vi "process_averager_imaq.vi"() -> ()   [LabVIEW 2011, in "Fiberscope_library.lvlib"]
uses:
  Fiberscope_library.lvlib
  typedefs/control_process_state_enum.ctl
  typedefs/control_process_state_cluster.ctl
  typedefs/feedback_from_process_enum.ctl
  typedefs/feedback_to_watchdog.ctl
  <vilib>/vision/Image Controls.llb/IMAQ Image.ctl
  typedefs/element_imaq_images_cluster.ctl
  <vilib>/vision/NI_Vision_Development_Module.lvlib
panel:
  out "Averages per frame":u8
  out "Average":u8
  out "error out":errorcluster
  in  "error in":errorcluster
  # "of"
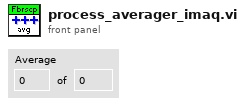
[diagram p1: front panel]
types:
  T1 = typedef "Fiberscope_library.lvlib/element_imaq_images_cluster.ctl" = cluster{"Images":T2[], "#channels":i32, "Last element?":bool}
  T2 = typedef "IMAQ Image.ctl" = refnum<image>
  T3 = typedef "Fiberscope_library.lvlib/feedback_to_watchdog.ctl" = cluster{"Feedback_from_process_enum":T4, "Process_name":string}
  T4 = typedef "Fiberscope_library.lvlib/feedback_from_process_enum.ctl" = enum16{"Has_initialised", "Changed_parameters", "Has_started", "Has_stopped", "Has_quitted", "Is_running", "Has_finished", "Custom"}
  T5 = typedef "Fiberscope_library.lvlib/control_process_state_cluster.ctl" = cluster{"Control_process_state_enum":T6, "variant":variant}
  T6 = typedef "Fiberscope_library.lvlib/control_process_state_enum.ctl" = enum16{"Init", "Quit", "Start", "Stop", "Change_parameters", "Running", "Finish", "Custom"}
  T7 = typedef "Image Type" = u32
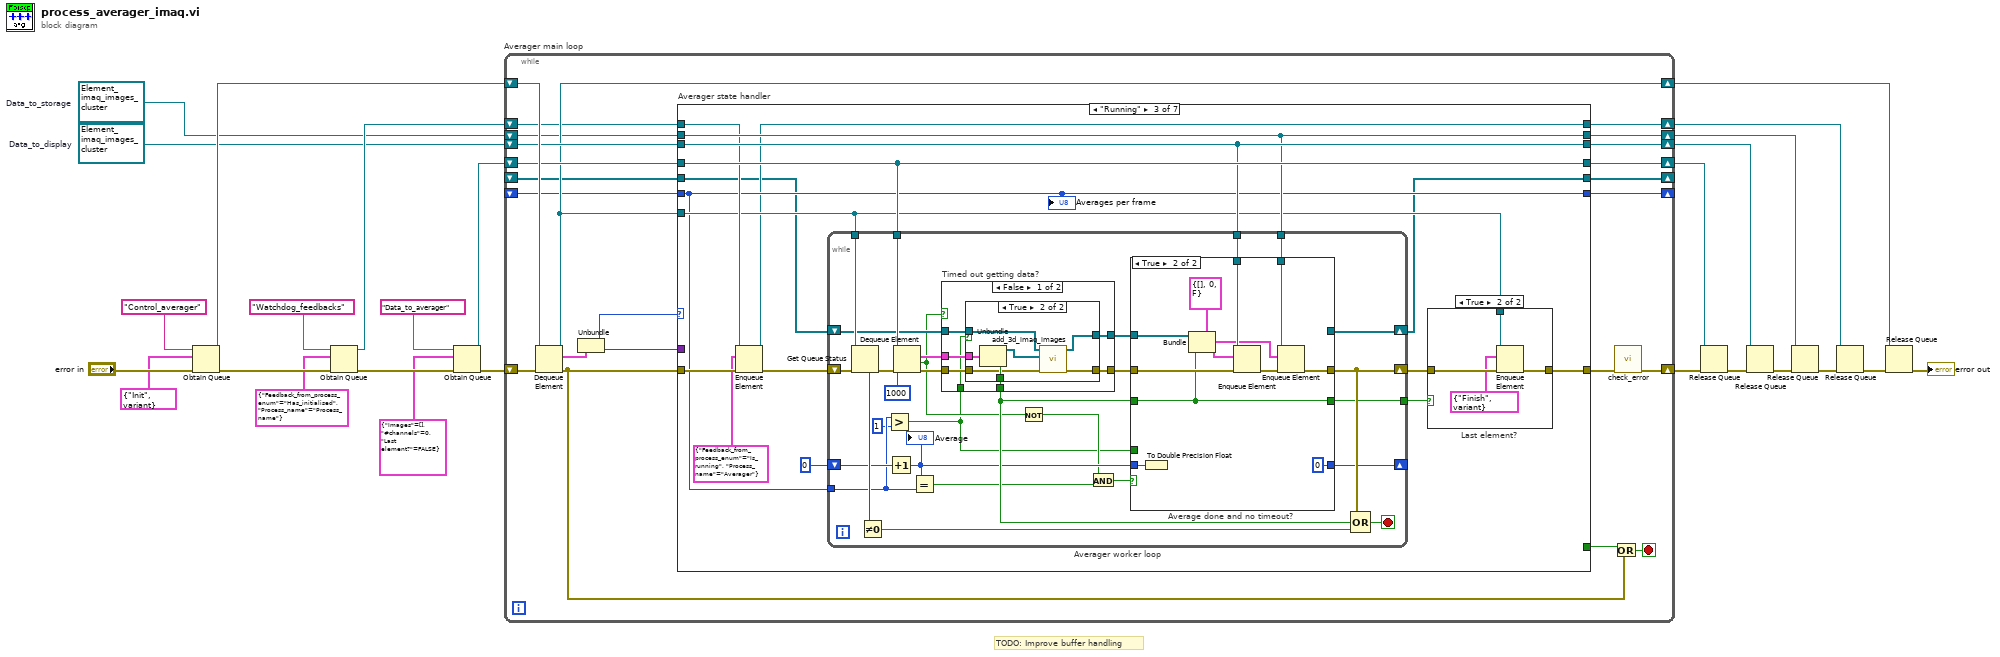
[diagram p0: block diagram]
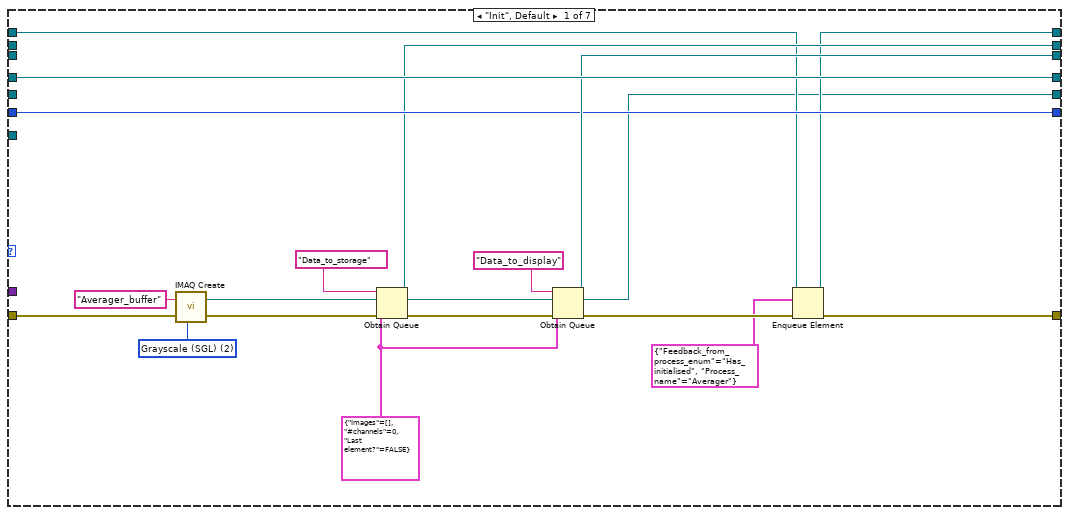
[diagram p2: hidden frame]
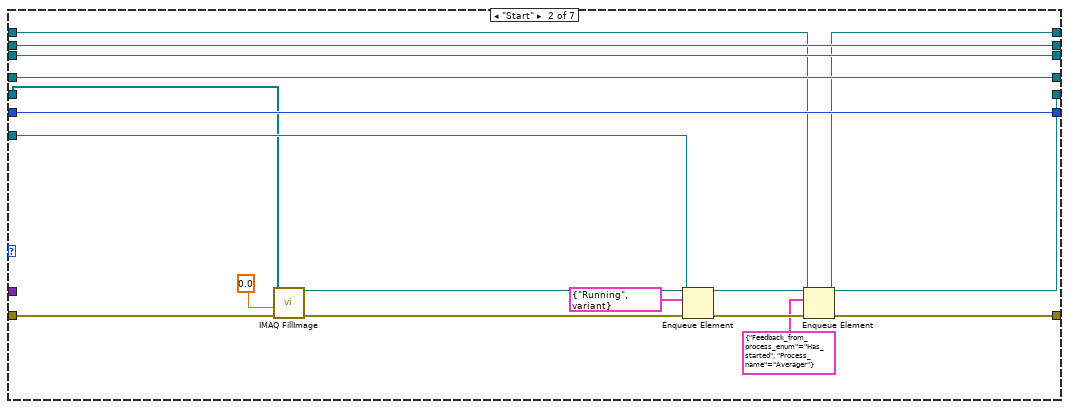
[diagram p3: hidden frame]
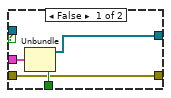
[diagram p6: hidden frame]
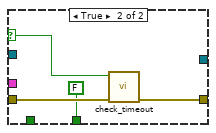
[diagram p7: hidden frame]
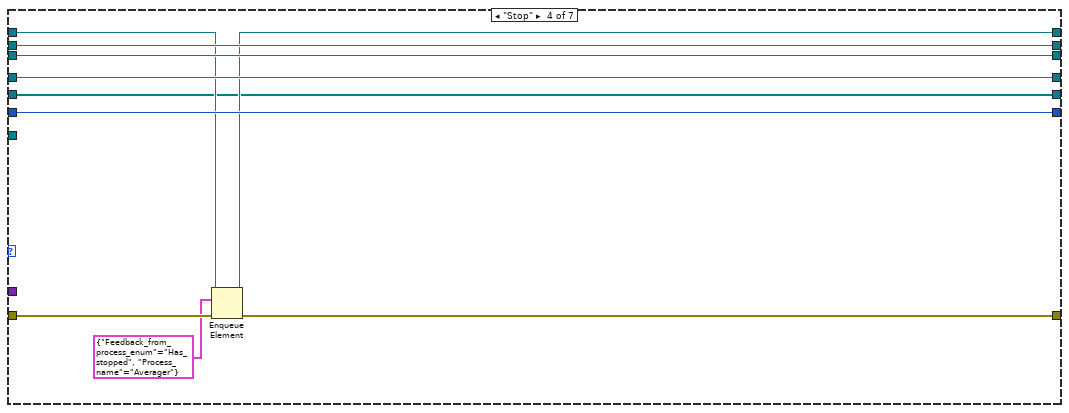
[diagram p8: hidden frame]
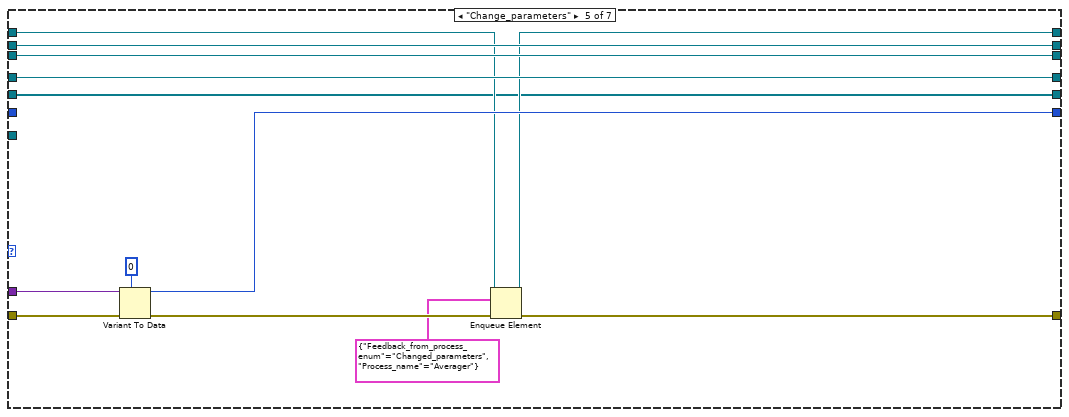
[diagram p9: hidden frame]
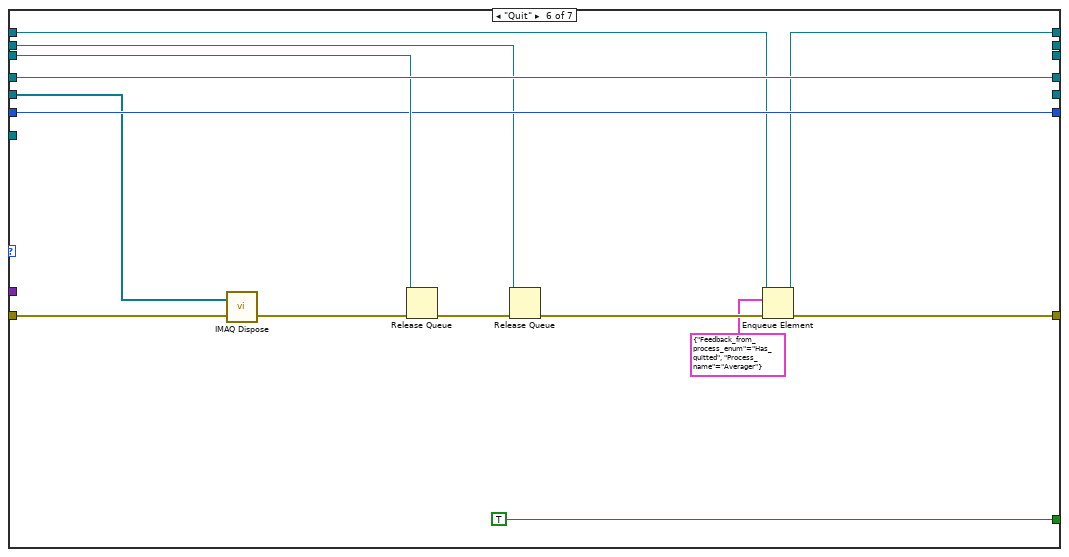
[diagram p10: hidden frame]
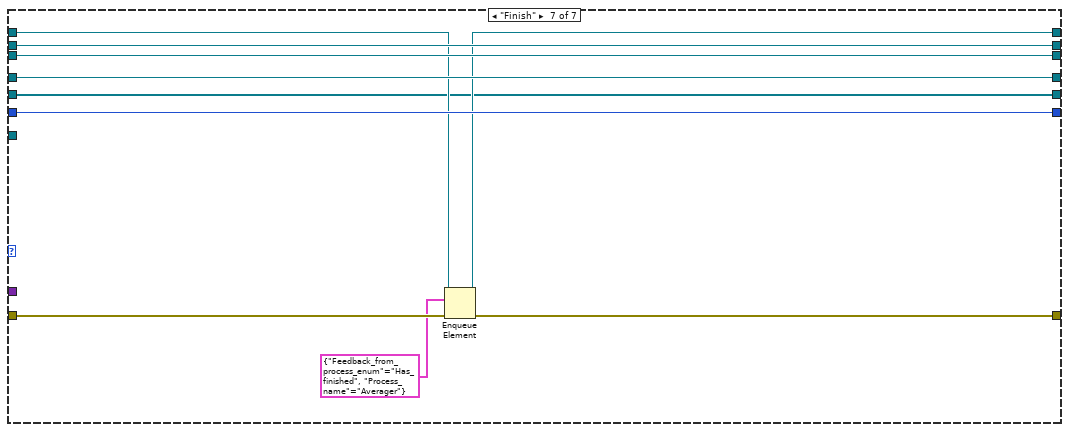
[diagram p11: hidden frame]
diagram:
  w1 = refnum<queue> refnum  # Data_to_display
  w2 = refnum<queue> refnum  # Data_to_storage
  # "TODO: Improve buffer handling"
  n1 = Obtain Queue(name (unnamed)="Control_averager", element data type=T5 {"Control_process_state_enum"=enum."Init", "variant"=variant} ("Control_process_state_cluster"), error in (no error)="error in") -> (queue out=w21:refnum<queue>, error out=w8:errorcluster)  [unwired: 2 in, 1 out]
  n2 = Obtain Queue(name (unnamed)="Watchdog_feedbacks", element data type=T3 {"Feedback_from_process_enum"=enum."Has_initialised", "Process_name"="Process_name"}, error in (no error)=w8) -> (queue out=w5:refnum<queue>, error out=w7:errorcluster)  [unwired: 2 in, 1 out]
  n3 = Obtain Queue(name (unnamed)="Data_to_averager", element data type=T1 {"Images"=[], "#channels"=0, "Last element?"=FALSE} ("Element_imaq_images_cluster"), error in (no error)=w7) -> (queue out=w20:refnum<queue>, error out=w22:errorcluster)  [unwired: 2 in, 1 out]
  n4 = while "Averager main loop" {
    shift-right: [w40] -> w19
    shift-left: w22 -> [w49]
    shift-right: [w37] -> w17
    shift-left: w21 -> [w48]
    shift-right: [w44] -> w18
    shift-left: w20 -> [w45]
    shift-right: [w42] -> w13
    shift-left: w1 -> [w43]
    shift-right: [w36] -> _
    shift-left: _ -> [w35]
    shift-right: [w33] -> w12
    shift-left: w2 -> [w34]
    shift-right: [w29] -> w9
    shift-left: w5 -> [w30]
    shift-right: [w28] -> _
    shift-left: _ -> [w27]
    stop <- w39 stop-if-true
    n5 = Dequeue Element(queue=w48, error in (no error)=w49) -> (queue out=w37:refnum<queue>, element=w47:T5, error out=w31:errorcluster)  [unwired: 1 in, 1 out]
    n6 = Unbundle(w47) -> ("Control_process_state_enum"=w46:T6, "variant"=w38:variant)
    n7 = case "Averager state handler" shown="\"Running\"" w46 {
      tunnel: w31 -> [w52 w72 w96 w176 w191 w196 w213]
      tunnel: [w59 w78 w92 w175 w185 w200 w212] -> w41
      tunnel: w45 -> [w67 w83 w99 w180 w193 w207 w217]
      tunnel: [w67 w83 w99 w180 w193 w207 w217] -> w44
      tunnel: w43 -> [_ w82 w98 w179 w192 w205 w216]
      tunnel: [w65 w82 w98 w179 w192 _ w216] -> w42
      tunnel: [_ _ _ _ _ TRUE _] -> w32
      tunnel: w38 -> [_ _ _ _ w190 _ _]
      tunnel: w37 -> [_ w77 w91 _ _ _ _]
      tunnel: [w64 w81 w89 w178 w189 w204 w215] -> w36
      tunnel: w35 -> [w64 w81 w89 w178 _ w204 w215]
      tunnel: w34 -> [_ w80 w97 w177 w188 w202 w214]
      tunnel: [w61 w80 w97 w177 w188 _ w214] -> w33
      tunnel: w30 -> [w58 w75 w94 w174 w184 w199 w211]
      tunnel: [w57 w74 w87 w173 w183 w198 w210] -> w29
      tunnel: [w50 w69 w84 w171 w181 _ w208] -> w28
      tunnel: w27 -> [_ w70 w85 w171 w181 w194 w208]
      frame "Init", Default {
        w53 = T7 2 items=["Grayscale (U8)", "Grayscale (I16)", "Grayscale (SGL)", "Complex (CSG)", "RGB (U32)", "HSL (U32)", "RGB (U64)", "Grayscale (U16)"] ("Image Type")
        w55 = T1 {"Images"=[], "#channels"=0, "Last element?"=FALSE} ("Element_imaq_images_cluster")
        n8 = call "IMAQ Create"("Image Name"="Averager_buffer", "Image Type"=w53, "error in (no error)"=w52) -> ("New Image"=w50:T2, "error out"=w51:errorcluster)  [unwired: 2 in]
        n9 = Obtain Queue(name (unnamed)="Data_to_storage", element data type=w55, error in (no error)=w51) -> (queue out=w61:refnum<queue>, error out=w62:errorcluster)  [unwired: 2 in, 1 out]
        n10 = Obtain Queue(name (unnamed)="Data_to_display", element data type=w55, error in (no error)=w62) -> (queue out=w65:refnum<queue>, error out=w60:errorcluster)  [unwired: 2 in, 1 out]
        n11 = Enqueue Element(queue=w58, element=T3 {"Feedback_from_process_enum"=enum."Has_initialised", "Process_name"="Averager"}, error in (no error)=w60) -> (queue out=w57:refnum<queue>, error out=w59:errorcluster)  [unwired: 1 in, 1 out]
      }
      frame "Start" {
        n12 = call "IMAQ FillImage"("error in (no error)"=w72, "Pixel Value (U8, U16, I16, Float)"=sgl 0.0, "Image"=w70) -> ("error out"=w71:errorcluster, "Image Out"=w69:T2)  [unwired: 7 in]
        n13 = Enqueue Element(queue=w77, element=T5 {"Control_process_state_enum"=enum."Running", "variant"=variant}, error in (no error)=w71) -> (error out=w79:errorcluster)  [unwired: 1 in, 2 out]
        n14 = Enqueue Element(queue=w75, element=T3 {"Feedback_from_process_enum"=enum."Has_started", "Process_name"="Averager"}, error in (no error)=w79) -> (queue out=w74:refnum<queue>, error out=w78:errorcluster)  [unwired: 1 in, 1 out]
      }
      frame "Running" {
        n15 = Enqueue Element(queue=w94, element=T3 {"Feedback_from_process_enum"=enum."Is_running", "Process_name"="Averager"}, error in (no error)=w96) -> (queue out=w87:refnum<queue>, error out=w95:errorcluster)  [unwired: 1 in, 1 out]
        n16 = while "Averager worker loop" {
          shift-right: [w116] -> w93
          shift-left: w95 -> [w133]
          tunnel: w91 -> [w132]
          tunnel: w99 -> [w131]
          tunnel: w98 -> [w129]
          tunnel: w97 -> [w127]
          shift-right: [w105] -> w84
          shift-left: w85 -> [w118]
          tunnel: w89 -> [w109]
          shift-right: [w115] -> _
          shift-left: u8 0 -> [w119]
          tunnel: [w110] -> w88
          stop <- w128 stop-if-true
          n17 = Get Queue Status(queue=w132, error in (no error)=w133) -> (error out=w125:errorcluster, # elements in queue=w121:i32)  [unwired: 1 in, 6 out]
          n18 = Not Equal To 0?(x=w121) -> (x != 0?=w120:bool)
          n19 = Greater?(x=w109, y=u8 1) -> (0:w107:bool)
          n20 = Increment(x=w119) -> (x+1=w117:u8)
          "Average" <- w117
          n21 = Dequeue Element(queue=w131, timeout in ms (-1)=1000, error in (no error)=w125) -> (element=w122:T1, timed out?=w112:bool, error out=w123:errorcluster)  [unwired: 1 out]
          n22 = Equal?(x=w117, y=w109) -> (x = y?=w114:bool)
          n23 = case "Timed out getting data?" shown="False" w112 {
            selector: w112 -> [_ w168]
            tunnel: w123 -> [w155 w170]
            tunnel: [w154 w169] -> w130
            tunnel: w122 -> [w152 _]
            tunnel: w118 -> [w153 _]
            tunnel: [w151 FALSE ("Last element?")] -> w126
            tunnel: w107 -> [w150 _]
            tunnel: [w149 _] -> w106
            frame False {
              n24 = case shown="True" w150 {
                tunnel: w155 -> [w157 w164]
                tunnel: [w157 w163] -> w154
                tunnel: w153 -> [_ w160]
                tunnel: w152 -> [w159 w166]
                tunnel: [w158 w165] -> w151
                tunnel: [w156 w162] -> w149
                frame False {
                  n25 = Unbundle(w159) -> ("Images"=w156:T2[], "Last element?"=w158:bool)  [unwired: 1 out]
                }
                frame True {
                  n26 = Unbundle(w166) -> ("Images"=w161:T2[], "Last element?"=w165:bool)  [unwired: 1 out]
                  n27 = call "add_3d_imaq_images.vi"("error in"=w164, "Images in 2"=w161, "Images in 1"=w160) -> ("error out"=w163:errorcluster, "Images out"=w162:T2[])  [unwired: 5 in]
                }
              }
            }
            frame True {
              n28 = call "check_timeout.vi"("error in"=w170, "Timeout?"=w168) -> ("error out"=w169:errorcluster)  [unwired: 9 in]
            }
          }
          n29 = Not(x=w112) -> (.not. x?=w111:bool)
          n30 = And(x=w111, y=w114) -> (x .and. y?=w113:bool)
          n31 = case "Average done and no timeout?" shown="True" w113 {
            tunnel: w130 -> [w137 w148]
            tunnel: w129 -> [_ w147]
            tunnel: [w137 w145] -> w116
            tunnel: w127 -> [_ w144]
            tunnel: w126 -> [w135 w140]
            tunnel: w117 -> [w136 w142]
            tunnel: [w136 u8 0 ("t")] -> w115
            tunnel: [w135 w140] -> w110
            tunnel: w107 -> [_ _]
            tunnel: w106 -> [w134 w138]
            tunnel: [w134 _] -> w105
            frame False {
            }
            frame True {
              n32 = To Double Precision Float(number=w142) -> ()  [unwired: 1 out]
              n33 = Bundle(cluster=T1 {"Images"=[], "#channels"=0, "Last element?"=FALSE} ("Element_imaq_images_cluster"), "Images"=w138, "Last element?"=w140) -> (w143:T1)  [unwired: 1 in]
              n34 = Enqueue Element(queue=w147, element=w143, error in (no error)=w148) -> (error out=w146:errorcluster)  [unwired: 1 in, 2 out]
              n35 = Enqueue Element(queue=w144, element=w143, error in (no error)=w146) -> (error out=w145:errorcluster)  [unwired: 1 in, 2 out]
            }
          }
          n36 = Compound Arithmetic op=OR(w116, w126, w120) -> (w128:bool)
        }
        n37 = case "Last element?" shown="True" w88 {
          tunnel: w93 -> [w100 w103]
          tunnel: [w100 w104] -> w92
          tunnel: w91 -> [_ w102]
          frame False {
          }
          frame True {
            n38 = Enqueue Element(queue=w102, element=T5 {"Control_process_state_enum"=enum."Finish", "variant"=variant} ("Control_process_state_cluster"), error in (no error)=w103) -> (error out=w104:errorcluster)  [unwired: 1 in, 2 out]
          }
        }
        "Averages per frame" <- w89
      }
      frame "Stop" {
        n39 = Enqueue Element(queue=w174, element=T3 {"Feedback_from_process_enum"=enum."Has_stopped", "Process_name"="Averager"}, error in (no error)=w176) -> (queue out=w173:refnum<queue>, error out=w175:errorcluster)  [unwired: 1 in, 1 out]
      }
      frame "Change_parameters" {
        n40 = Variant To Data(error in=w191, type=u8 0 ("Averages per frame"), Variant=w190) -> (data=w189:u8, error out=w186:errorcluster)
        n41 = Enqueue Element(queue=w184, element=T3 {"Feedback_from_process_enum"=enum."Changed_parameters", "Process_name"="Averager"}, error in (no error)=w186) -> (queue out=w183:refnum<queue>, error out=w185:errorcluster)  [unwired: 1 in, 1 out]
      }
      frame "Quit" {
        n42 = call "IMAQ Dispose"("Image"=w194, "error in (no error)"=w196) -> ("error out"=w195:errorcluster)  [unwired: 4 in]
        n43 = Release Queue(queue=w205, error in (no error)=w195) -> (error out=w203:errorcluster)  [unwired: 1 in, 2 out]
        n44 = Release Queue(queue=w202, error in (no error)=w203) -> (error out=w201:errorcluster)  [unwired: 1 in, 2 out]
        n45 = Enqueue Element(queue=w199, element=T3 {"Feedback_from_process_enum"=enum."Has_quitted", "Process_name"="Averager"}, error in (no error)=w201) -> (queue out=w198:refnum<queue>, error out=w200:errorcluster)  [unwired: 1 in, 1 out]
      }
      frame "Finish" {
        n46 = Enqueue Element(queue=w211, element=T3 {"Feedback_from_process_enum"=enum."Has_finished", "Process_name"="Averager"}, error in (no error)=w213) -> (queue out=w210:refnum<queue>, error out=w212:errorcluster)  [unwired: 1 in, 1 out]
      }
    }
    n47 = Or(x=w32, y=w31) -> (x .or. y?=w39:bool)
    n48 = call "check_error.vi"("error in"=w41) -> ("error out"=w40:errorcluster)  [unwired: 10 in]
  }
  n49 = Release Queue(queue=w18, error in (no error)=w19) -> (error out=w15:errorcluster)  [unwired: 1 in, 2 out]
  n50 = Release Queue(queue=w13, error in (no error)=w15) -> (error out=w14:errorcluster)  [unwired: 1 in, 2 out]
  n51 = Release Queue(queue=w12, error in (no error)=w14) -> (error out=w11:errorcluster)  [unwired: 1 in, 2 out]
  n52 = Release Queue(queue=w9, error in (no error)=w11) -> (error out=w10:errorcluster)  [unwired: 1 in, 2 out]
  n53 = Release Queue(queue=w17, error in (no error)=w10) -> (error out=→"error out":errorcluster)  [unwired: 1 in, 2 out]
